vi "TCP_FGV.vi"(0 "Command":string, 3 "error in (no error)":errorcluster, 4 "Operation":T1) -> (7 "Data Out":string, 10 "error out":errorcluster)   [LabVIEW 2021]
uses:
  TCP_FGV.ctl
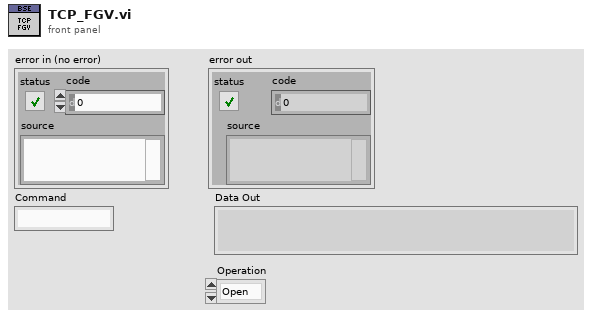
[diagram p1: front panel]
types:
  T1 = typedef "TCP_FGV.ctl" = enum16{"Open", "Read", "Write", "Close"}
  T2 = enum16{"Standard", "Buffered", "CRLF", "Immediate"}
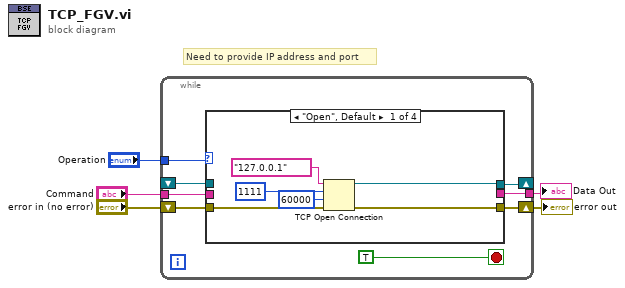
[diagram p0: block diagram]
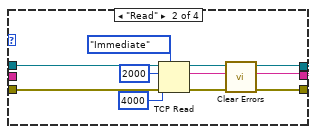
[diagram p2: hidden frame]
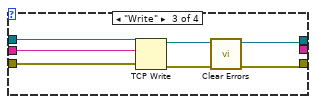
[diagram p3: hidden frame]
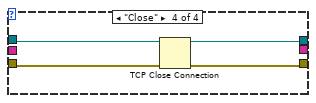
[diagram p4: hidden frame]
diagram:
  # "Need to provide IP address and port"
  n1 = while {
    shift-right: [w10] -> w3
    shift-left: "error in (no error)" -> [w11]
    shift-right: [w9] -> _
    shift-left: _ -> [w8]
    tunnel: "Operation" -> [w12]
    tunnel: [w7] -> w2
    tunnel: "Command" -> [w6]
    stop <- TRUE stop-if-true
    n2 = case shown="\"Open\", Default" w12 {
      tunnel: w11 -> [w19 w28 w34 w38]
      tunnel: [w18 w20 w29 w37] -> w10
      tunnel: [w14 w26 w30 w35] -> w9
      tunnel: w8 -> [_ w25 w31 w36]
      tunnel: [_ w24 _ _] -> w7
      tunnel: w6 -> [_ _ w32 _]
      frame "Open", Default {
        n3 = TCP Open Connection(address="127.0.0.1", remote port or service name=u16 1111, timeout ms (60000)=60000, error in (no error)=w19) -> (connection ID=w14:refnum<k5>, error out=w18:errorcluster)  [unwired: 1 in]
      }
      frame "Read" {
        n4 = TCP Read(connection ID=w25, bytes to read=2000, error in (no error)=w28, 7:T2."Immediate" ("mode (standard)"), 9:4000 ("timeout ms (25000)")) -> (connection ID out=w26:refnum<k5>, data out=w24:string, error out=w27:errorcluster)
        n5 = call <vilib>:"Clear Errors.vi"("error in (no error)"=w27) -> ("error out"=w20:errorcluster)  [unwired: 5 in, 1 out]
      }
      frame "Write" {
        n6 = TCP Write(connection ID=w31, data in=w32, error in (no error)=w34) -> (connection ID out=w30:refnum<k5>, error out=w33:errorcluster)  [unwired: 1 in, 1 out]
        n7 = call <vilib>:"Clear Errors.vi"("error in (no error)"=w33) -> ("error out"=w29:errorcluster)  [unwired: 5 in, 1 out]
      }
      frame "Close" {
        n8 = TCP Close Connection(connection ID=w36, error in (no error)=w38) -> (connection ID out=w35:refnum<k5>, error out=w37:errorcluster)  [unwired: 1 in]
      }
    }
  }
  "error out" <- w3
  "Data Out" <- w2
